vi "Set PDOs mapping.vi"(7 "timeout (1s)":dbl=1.0 min=0.0, 8 "error in (no error)":errorcluster, 11 "SDO object in":refnum<k20>) -> (0 "error out":errorcluster, 1 "completion codes":u32[](array[numeric]), 3 "SDO object out":refnum<k20>)   [LabVIEW 2016]
uses:
  Transmit PDO mapping.ctl
  Receive PDOs mapping.ctl
  Set PDO recive mapping.vi
  Set PDO transmit mapping.vi
  <vilib>/CANopenLib/CANOPEN.llb/CANopen SDO Write [U8].vi
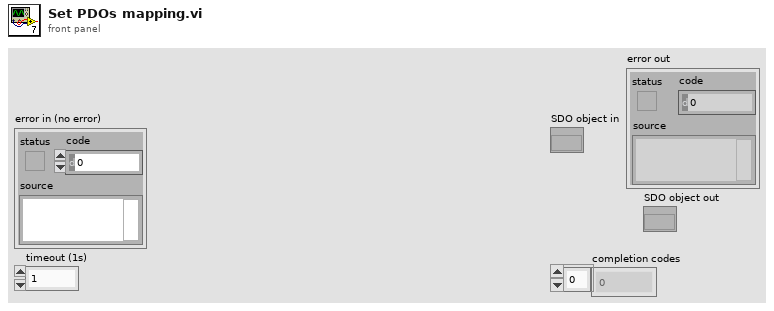
[diagram p1: front panel]
types:
  T1 = typedef "Receive PDOs mapping.ctl" = cluster{"General state":cluster{"Statusword":u32, "Motor temperature":u32, "Controller temperature":u32}, "Errors":cluster{"Error register":u32, "Error code":u32, "Warnings":u32}, "Traction indicators":cluster{"Velocity actual value":u32, "Troque actual value":u32, "Electric power":u32, "DC current":u32}, "Others":cluster{"Phase A current":u32, "Phase B current":u32, "Current demand":u32}}
  T2 = typedef "Transmit PDO mapping.ctl" = cluster{"Maximum controller current":u32, "Target torque":u32, "Target velocity":u32}
  T3 = cluster{"Statusword":u32, "Motor temperature":u32, "Controller temperature":u32}
  T4 = cluster{"Error register":u32, "Error code":u32, "Warnings":u32}
  T5 = cluster{"Velocity actual value":u32, "Troque actual value":u32, "Electric power":u32, "DC current":u32}
  T6 = cluster{"Phase A current":u32, "Phase B current":u32, "Current demand":u32}
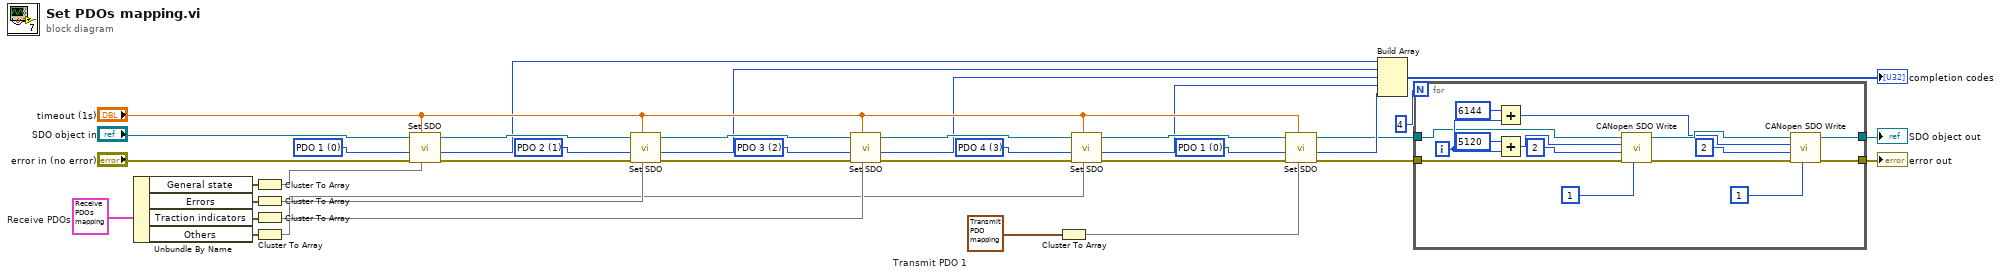
[diagram p0: block diagram]
diagram:
  w24 = u8 0 items=["PDO 1", "PDO 2", "PDO 3", "PDO 4"] ("PDO channel")
  w27 = u8 3 items=["PDO 1", "PDO 2", "PDO 3", "PDO 4"] ("PDO channel")
  w30 = u8 2 items=["PDO 1", "PDO 2", "PDO 3", "PDO 4"] ("PDO channel")
  w31 = u8 1 items=["PDO 1", "PDO 2", "PDO 3", "PDO 4"] ("PDO channel")
  w32 = u8 0 items=["PDO 1", "PDO 2", "PDO 3", "PDO 4"] ("PDO channel")
  w35 = T1 {"General state"={"Statusword"=1614872592, "Motor temperature"=539295752, "Controller temperature"=539361288}, "Errors"={"Error register"=268501000, "Error code"=1614741520, "Warnings"=539426832}, "Traction indicators"={"Velocity actual value"=1617690656, "Troque actual value"=1618411536, "Electric power"=539230240, "DC current"=539164704}, "Others"={"Phase A current"=537853968, "Phase B current"=537919504, "Current demand"=538574864}}  # Receive PDOs
  w34 = T2 {"Maximum controller current"=542113824, "Target torque"=1618018320, "Target velocity"=1627324448}  # Transmit PDO 1
  n1 = Unbundle By Name(w35) -> ("General state"=w38:T3, "Errors"=w37:T4, "Traction indicators"=w36:T5, "Others"=w26:T6)
  n2 = Cluster To Array(cluster=w38) -> (array=w33:u32[])
  n3 = Cluster To Array(cluster=w37) -> (array=w29:u32[])
  n4 = Cluster To Array(cluster=w36) -> (array=w28:u32[])
  n5 = Cluster To Array(cluster=w26) -> (array=w25:u32[])
  n6 = call-poly "Set SDO.vi"("PDO mapping"=w33, "timeout (1s)"="timeout (1s)", "error in (no error)"="error in (no error)", "PDO channel"=w32, "SDO object in"="SDO object in") -> ("error out"=w13:errorcluster, "completion code"=w11:u32, "SDO object out"=w20:refnum<k20>)  [unwired: 4 in]
  n7 = call-poly "Set SDO.vi"("PDO mapping"=w29, "timeout (1s)"="timeout (1s)", "error in (no error)"=w13, "PDO channel"=w31, "SDO object in"=w20) -> ("error out"=w14:errorcluster, "completion code"=w10:u32, "SDO object out"=w19:refnum<k20>)  [unwired: 4 in]
  n8 = call-poly "Set SDO.vi"("PDO mapping"=w28, "timeout (1s)"="timeout (1s)", "error in (no error)"=w14, "PDO channel"=w30, "SDO object in"=w19) -> ("error out"=w15:errorcluster, "completion code"=w9:u32, "SDO object out"=w18:refnum<k20>)  [unwired: 4 in]
  n9 = Cluster To Array(cluster=w34) -> (array=w23:u32[])
  n10 = call-poly "Set SDO.vi"("PDO mapping"=w25, "timeout (1s)"="timeout (1s)", "error in (no error)"=w15, "PDO channel"=w27, "SDO object in"=w18) -> ("error out"=w16:errorcluster, "completion code"=w8:u32, "SDO object out"=w17:refnum<k20>)  [unwired: 4 in]
  n11 = call-poly "Set SDO.vi"("PDO mapping"=w23, "timeout (1s)"="timeout (1s)", "error in (no error)"=w16, "PDO channel"=w24, "SDO object in"=w17) -> ("error out"=w3:errorcluster, "completion code"=w7:u32, "SDO object out"=w4:refnum<k20>)  [unwired: 4 in]
  n12 = Build Array(w11, w10, w9, w8, w7) -> (→"completion codes":u32[])
  n13 = for {
    N: 4 -> [_]
    tunnel: w4 -> [w42]
    tunnel: w3 -> [w41]
    tunnel: [w40] -> w2
    tunnel: [w39] -> w1
    i -> [w43]
    n14 = Add(x=u16 6144 ("object index"), y=w43) -> (x+y=w45:i32)
    n15 = Add(x=u16 5120 ("object index"), y=w43) -> (x+y=w46:i32)
    n16 = call-poly <vilib>:"CANopen SDO Write.vi"("U8 data"=u8 1 ("object index"), "error in (no error)"=w41, "object sub-index (0)"=u8 2 ("object index"), "object index"=w46, "SDO object in"=w42) -> ("error out"=w49:errorcluster, "SDO object out"=w48:refnum<k20>)  [unwired: 4 in, 1 out]
    n17 = call-poly <vilib>:"CANopen SDO Write.vi"("U8 data"=u8 1 ("object index"), "error in (no error)"=w49, "object sub-index (0)"=u8 2 ("object index"), "object index"=w45, "SDO object in"=w48) -> ("error out"=w39:errorcluster, "SDO object out"=w40:refnum<k20>)  [unwired: 4 in, 1 out]
  }
  "SDO object out" <- w2
  "error out" <- w1
